vi "ECUSignalSender_Create.vi"() -> (14 "EventHandl(订阅事件用)":refnum<event-registration>[](array[refnum]), 15 "SMOArry":refnum<class "SignalSenderLoop.lvclass">[](array[class]), 19 "错误输出":errorcluster)   [LabVIEW 2020]
uses:
  Typedefs/PublicEvents--Cluster.ctl
  Typedefs/SetpointChanged--EventData--Cluster.ctl
  Typedefs/Data.ctl
  <vilib>/JKI/JKI SMO/SMO/Typedefs/Public Events.ctl
  <vilib>/JKI/JKI SMO/SMO/Typedefs/SMOState --Enum.ctl
  <vilib>/JKI/JKI SMO/SMO/Typedefs/Reserve State--Enum.ctl
  SignalSenderLoop.lvclass
  C:/Program Files (x86)/National Instruments/LabVIEW 2020/vi.lib/JKI/JKI SMO/SMO/SMO.lvclass
  <vilib>/JKI/JKI SMO/SMO/SMO.lvclass/SMO.ctl
  <vilib>/JKI/JKI SMO/SMO/Private/ReftoDVR--SMO.vi
  <vilib>/JKI/JKI SMO/SMO/SMO.lvclass
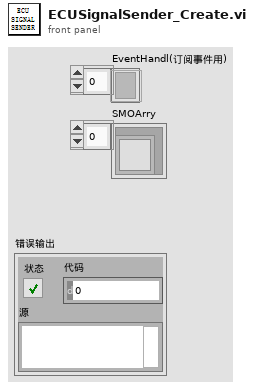
[diagram p1: front panel]
types:
  T1 = typedef "SignalSenderLoop.lvclass/SignalFrameSet.ctl" = cluster{"Port_No.":refnum<k21>, "计数Count":bool, "校验CheckSum":bool, "MessageFrame":refnum<k21>, "校验算法名称":string}
  T2 = typedef "SMO.lvclass/Public Events.ctl" = cluster{"Error":refnum<user-event>, "State":refnum<user-event>, "Reserve State":refnum<user-event>}
  T3 = typedef "SignalSenderLoop.lvclass/PublicEvents--Cluster.ctl" = cluster{"Setpoint Changed":refnum<user-event>, "Value Changed":refnum<user-event>}
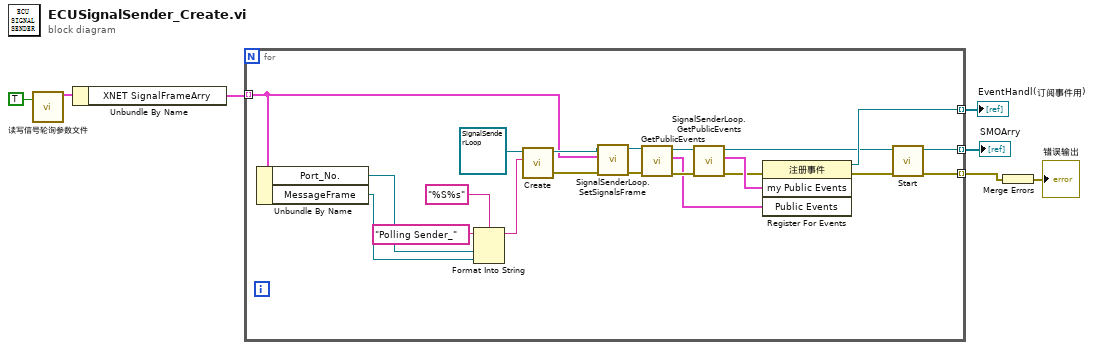
[diagram p0: block diagram]
diagram:
  n1 = call "读写信号轮询参数文件.vi"("T:Read/F:Write"=TRUE) -> ("信号轮询发送设置Out"=w6:cluster{"XNET SignalFrameArry":T1[]})  [unwired: 17 in, 1 out]
  n2 = Unbundle By Name(w6) -> ("XNET SignalFrameArry"=w5:T1[])
  n3 = for {
    tunnel: w5 -> [w10] mode=indexing
    tunnel: [w15] -> w4 mode=indexing
    tunnel: [w12] -> w3 mode=indexing
    tunnel: [w11] -> w2 mode=indexing
    n4 = Unbundle By Name(w10) -> ("Port_No."=w9:refnum<k21>, "MessageFrame"=w8:refnum<k21>)
    n5 = Format Into String(format string="%S%s" ("格式字符串"), initial string="Polling Sender_", w9, w8) -> (resulting string=w16:string)  [unwired: 1 in, 1 out]
    n6 = call <vilib>:"Create.vi"("Subsystem Name (optional)"=w16, "SMO"=refnum<class "SignalSenderLoop.lvclass"> refnum ("SMO.Template.lvclass")) -> ("error out"=w18:errorcluster, "SMO out"=w20:refnum<class "SignalSenderLoop.lvclass">)  [unwired: 7 in, 1 out]
    n7 = call "SignalSenderLoop.SetSignalsFrame.vi"("error in (no error)"=w18, "SignalFrameSet"=w10, "SignalSenderLoop"=w20) -> ("error out"=w17:errorcluster, "SignalSenderLoop out"=w19:refnum<class "SignalSenderLoop.lvclass">)  [unwired: 7 in]
    n8 = call <vilib>:"GetPublicEvents.vi"("error in (no error)"=w17, "SMO"=w19) -> ("error out"=w24:errorcluster, "Public Events"=w21:T2, "SMO out"=w23:refnum<class "SignalSenderLoop.lvclass">)  [unwired: 7 in]
    n9 = call "SignalSenderLoop.GetPublicEvents.vi"("error in (no error)"=w24, "SignalSenderLoop"=w23) -> ("error out"=w22:errorcluster, "my Public Events"=w25:T3, "SignalSenderLoop out"=w14:refnum<class "SignalSenderLoop.lvclass">)  [unwired: 7 in]
    n10 = register-events(error in=w22, w25, w21) -> (reference out=w15:refnum<event-registration>, error out=w13:errorcluster)  [unwired: 1 in]
    n11 = call <vilib>:"Start.vi"("error in (no error)"=w13, "SMO"=w14) -> ("error out"=w11:errorcluster, "SMO out"=w12:refnum<class "SignalSenderLoop.lvclass">)  [unwired: 8 in]
  }
  "EventHandl(订阅事件用)" <- w4
  "SMOArry" <- w3
  n12 = Merge Errors(w2) -> (→"错误输出":errorcluster)
